vi "Pasco Zero Out.vi"(0 "LDrive Distance":dbl, 5 "RDrive Distance":dbl, 7 "Gyro Heading":dbl, 9 "Zero Out Distance":bool, 11 "Zero Out Gyro":bool) -> (4 "LDrive Distance":dbl, 6 "RDrive Distance":dbl, 8 "Gyro Heading":dbl)   [LabVIEW 2011]
panel:
  out "Gyro Negated":dbl
  out "RDrive Negated":dbl
  out "LDrive Negated":dbl
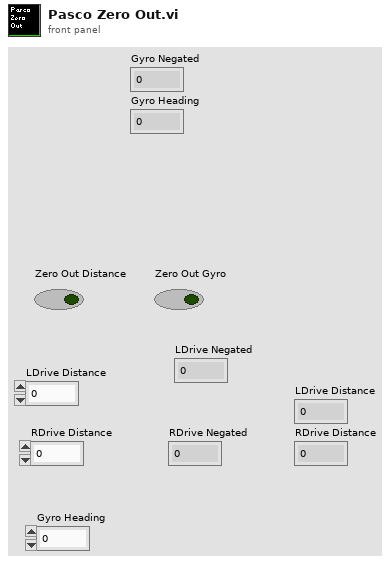
[diagram p1: front panel]
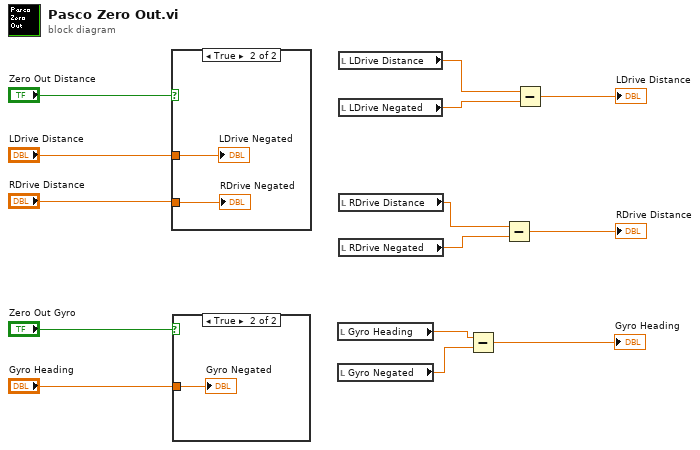
[diagram p0: block diagram]
diagram:
  n1 = case shown="True" "Zero Out Distance" {
    tunnel: "LDrive Distance" -> [_ w16]
    tunnel: "RDrive Distance" -> [_ w15]
    frame False {
    }
    frame True {
      "LDrive Negated" <- w16
      "RDrive Negated" <- w15
    }
  }
  n2 = case shown="True" "Zero Out Gyro" {
    tunnel: "Gyro Heading" -> [_ w17]
    frame False {
    }
    frame True {
      "Gyro Negated" <- w17
    }
  }
  n3 = local read "Gyro Heading"() -> (w3:dbl)
  n4 = local read "Gyro Negated"() -> (w2:dbl)
  n5 = local read "LDrive Distance"() -> (w9:dbl)
  n6 = local read "LDrive Negated"() -> (w10:dbl)
  n7 = local read "RDrive Distance"() -> (w8:dbl)
  n8 = local read "RDrive Negated"() -> (w11:dbl)
  n9 = Subtract(x=w3, y=w2) -> (x-y=→"Gyro Heading":dbl)
  n10 = Subtract(x=w8, y=w11) -> (x-y=→"RDrive Distance":dbl)
  n11 = Subtract(x=w9, y=w10) -> (x-y=→"LDrive Distance":dbl)
